vi "GetControl_PageSelector.vi"(7 "Control Class":refnum<vi>, 8 "error in (no error)":errorcluster, 10 "Control Label":string, 11 "CtlLookup In":T1) -> (0 "error out":errorcluster, 2 "Reference Out":refnum<vi>, 3 "CtlLookup Out":T1)   [LabVIEW 2018, in "CtlReferences.lvlib" / "CtlReferences.lvclass"]
uses:
  CtlReferences.lvclass
  TypeDefs/CtlLookup.ctl
  CtlReferences.lvclass/CtlReferences.ctl
  GetCtlRef_Lookup.vi
  <vilib>/Utility/error.llb/Error Cluster From Error Code.vi
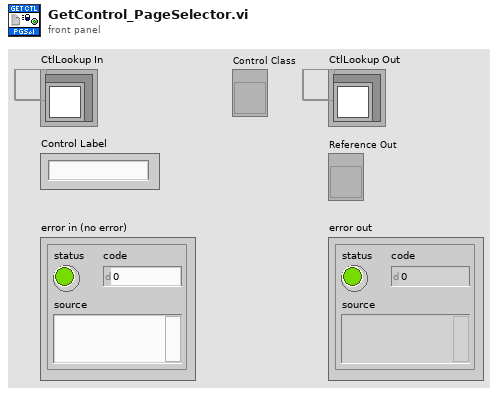
[diagram p1: front panel]
types:
  T1 = typedef "CtlReferences.lvlib/CtlReferences.lvclass/CtlLookup.ctl" = refnum<data-value>
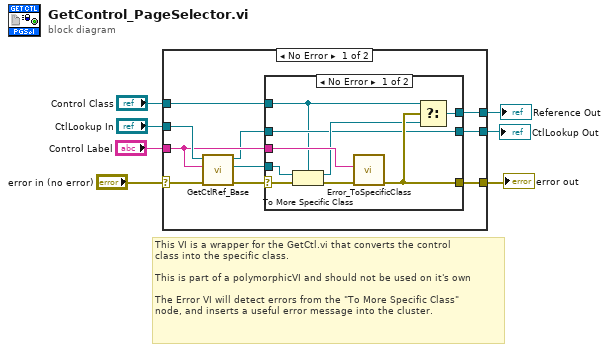
[diagram p0: block diagram]
diagram:
  # "This VI is a wrapper for the GetCtl.vi that converts the control\nclass into the specific class.\n\nThis is part of a polymorphicVI and should not be used on it's own\n\nThe Error VI will detect errors from the \"To More Specific Class\" \nnode, and inserts a useful error message into the cluster."
  n1 = case shown="No Error" "error in (no error)" {
    selector: "error in (no error)" -> [w11 w30]
    tunnel: [w15 w30] -> w6
    tunnel: "CtlLookup In" -> [w14 w32]
    tunnel: [w8 w32] -> w4
    tunnel: [w13 w31] -> w3
    tunnel: "Control Class" -> [w12 w31]
    tunnel: "Control Label" -> [w10 _]
    frame No Error {
      n2 = call "GetCtlRef_Base.vi"("error in (no error)"=w11, "Control Label"=w10, "CtlLookup In"=w14) -> ("error out"=w16:errorcluster, "CtlRef Out"=w17:refnum<vi>, "CtlLookup Out"=w9:T1)  [unwired: 6 in]
      n3 = case shown="No Error" w16 {
        selector: w16 -> [w25 w29]
        tunnel: w17 -> [w26 _]
        tunnel: [w22 w29] -> w15
        tunnel: w10 -> [w23 _]
        tunnel: [w20 w28] -> w13
        tunnel: w12 -> [w18 w28]
        tunnel: w9 -> [w19 w27]
        tunnel: [w19 w27] -> w8
        frame No Error {
          n4 = To More Specific Class(target class=w18, reference=w26, error in=w25) -> (specific class reference=w21:refnum<vi>, error out=w24:errorcluster)
          n5 = call "Error_ToSpecificClass.vi"("error in (no error)"=w24, "Control Label"=w23) -> ("error out"=w22:errorcluster)  [unwired: 9 in]
          n6 = Select(t=w18, s=w22, f=w21) -> (s? t:f=w20:refnum<vi>)
        }
        frame Error {
        }
      }
    }
    frame Error {
    }
  }
  "error out" <- w6
  "CtlLookup Out" <- w4
  "Reference Out" <- w3
